vi "Bulk Add DO Coil Dialog.vi"(8 "error in (no error)":errorcluster, 10 "Starting Address":u16) -> (0 "error out":errorcluster, 1 "Cancelled?":bool, 2 "Quantity Out":u16, 3 "Root Name Out":string, 5 "Starting Address Out":u16)   [LabVIEW 2021]
panel:
  in  "Cancel Button":bool
  in  "OK Button":bool
  in  "Quantity":u16
  in  "Root Name":string="Coil"
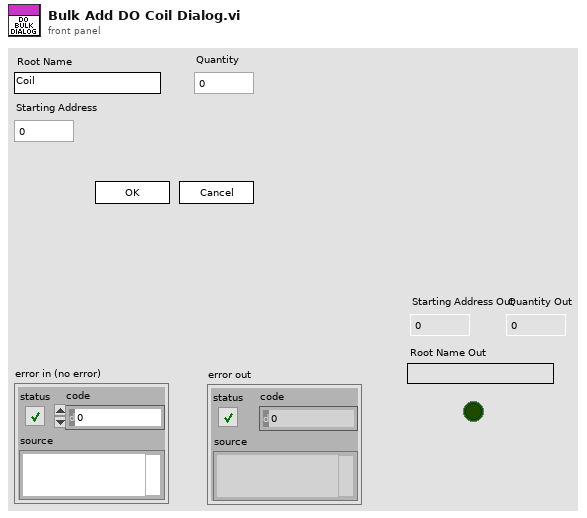
[diagram p1: front panel]
types:
  T1 = enum32{"Invalid", "Standard", "Closed", "Hidden", "Minimized", "Maximized"}
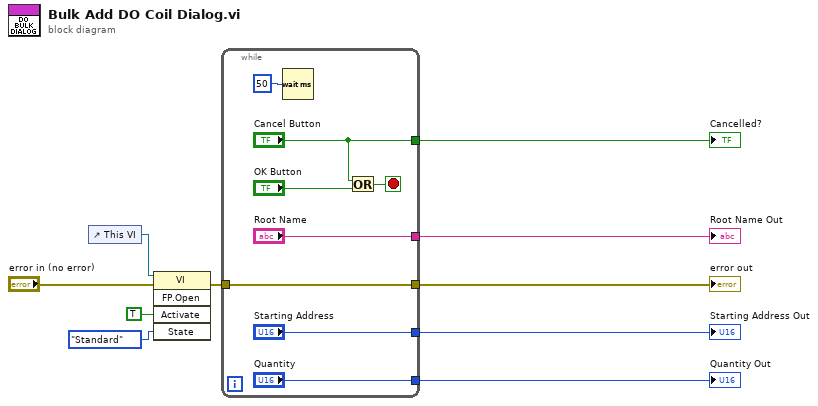
[diagram p0: block diagram]
diagram:
  n1 = control-ref of="This VI"() -> (w6:refnum<vi>)
  n2 = invoke class="VI" method="FP.Open"(reference=w6, error in="error in (no error)", "Activate"=TRUE ("Activate?"), "State"=T1."Standard") -> (error out=w1:errorcluster)  [unwired: 1 in, 4 out]
  n3 = while {
    tunnel: ["Cancel Button"] -> w10
    tunnel: ["Root Name"] -> w9
    tunnel: ["Quantity"] -> w8
    tunnel: ["Starting Address"] -> w7
    tunnel: [w11] -> w2
    tunnel: w1 -> [w11]
    stop <- w17 stop-if-true
    n4 = Wait (ms)(milliseconds to wait=u32 50) -> ()  [unwired: 1 out]
    n5 = Or(x="Cancel Button", y="OK Button") -> (x .or. y?=w17:bool)
  }
  "error out" <- w2
  "Root Name Out" <- w9
  "Starting Address Out" <- w7
  "Cancelled?" <- w10
  "Quantity Out" <- w8
